vi "Set Master or Slave.vi"(8 "error in (no error)":errorcluster, 10 "Master/Slave":enum32{"Master", "Slave"}(ring), 11 "Controller UI in":refnum<class "Controller UI.lvclass">) -> (0 "error out":errorcluster, 3 "Controller UI out":refnum<class "Controller UI.lvclass">)   [LabVIEW 2016, in "Controller UI.lvlib" / "Controller UI.lvclass"]
uses:
  <userlib>/Common Components/Controller UI/Controller UI.lvclass
  <userlib>/Common Components/Controller UI/Controller UI.lvclass/Controller UI.ctl
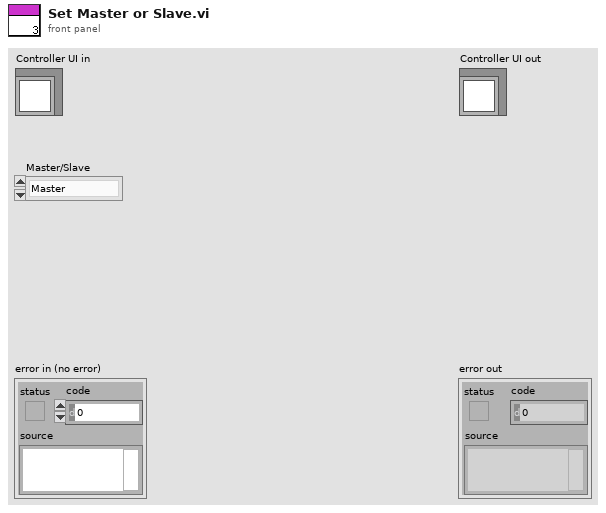
[diagram p1: front panel]
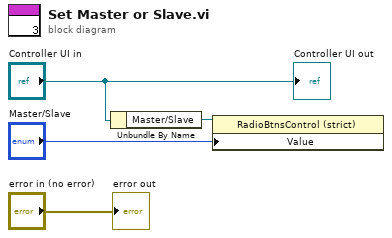
[diagram p0: block diagram]
diagram:
  n1 = Unbundle By Name("Controller UI in") -> ("Master/Slave"=w2:refnum<vi>)
  n2 = property class="RadioBtnsControl (strict)"(reference=w2, "Value"="Master/Slave") -> ()  [unwired: 1 in, 2 out]
  "error out" <- "error in (no error)"
  "Controller UI out" <- "Controller UI in"
